vi "Set Column Widths (Pixels).vi"(8 "error in (no error)":errorcluster, 10 "Column Widths [pixels]":u32[](array[numeric]), 11 "MulticolumnListbox in":refnum<vi>) -> (0 "error out":errorcluster)   [LabVIEW 2020, in "ListboxExtensions.lvlib"]
doc: "设置列宽（像素）"
uses:
  ListboxExtensions.lvlib
  <vilib>/Utility/miscctls.llb/LVRowAndColumnTypeDef.ctl
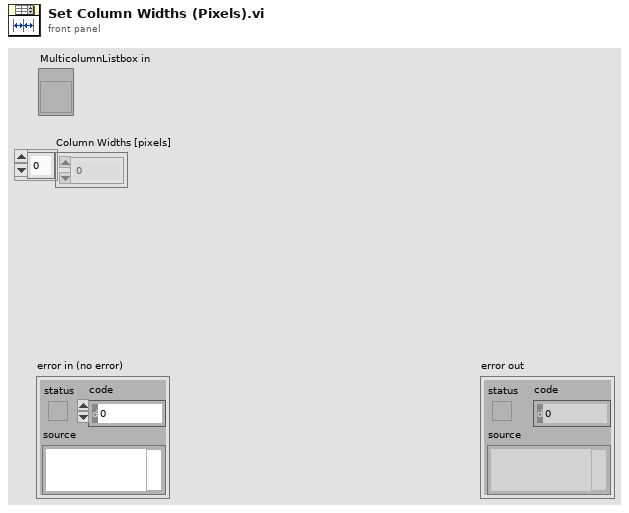
[diagram p1: front panel]
types:
  T1 = typedef "LVRowAndColumnTypeDef.ctl" = cluster{"Row":i32, "Column":i32}
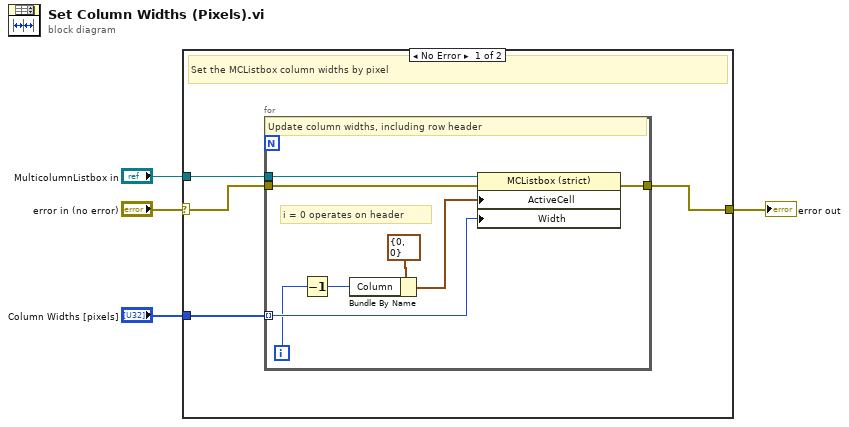
[diagram p0: block diagram]
diagram:
  n1 = case shown="No Error" "error in (no error)" {
    selector: "error in (no error)" -> [w6 w17]
    tunnel: "Column Widths [pixels]" -> [w8 _]
    tunnel: "MulticolumnListbox in" -> [w7 _]
    tunnel: [w5 w17] -> w1
    frame No Error {
      # "Set the MCListbox column widths by pixel"
      n2 = for {
        tunnel: [w16] -> w5
        tunnel: w7 -> [w15]
        tunnel: w8 -> [w12] mode=indexing
        tunnel: w6 -> [w10]
        i -> [w9]
        # "i = 0 operates on header"
        # "Update column widths, including row header"
        n3 = Decrement(x=w9) -> (x-1=w11:i32)
        n4 = Bundle By Name(cluster=T1 {"Row"=0, "Column"=0} ("Active Cell:Active Cell"), "Column"=w11) -> (w13:T1)
        n5 = property class="MCListbox (strict)"(reference=w15, error in=w10, "ActiveCell"=w13, "Width"=w12) -> (error out=w16:errorcluster)  [unwired: 1 out]
      }
    }
    frame Error {
      # "Do nothing to the MCListbox if error in"
    }
  }
  "error out" <- w1
